vi "Read String in A.vi"(8 "error in (no error)":errorcluster, 11 "A in":refnum<class "A.lvclass">) -> (0 "error out":errorcluster, 2 "String in A":string, 3 "A out":refnum<class "A.lvclass">)   [LabVIEW 2013, in "A.lvclass"]
uses:
  A.lvclass
  A.lvclass/A.ctl
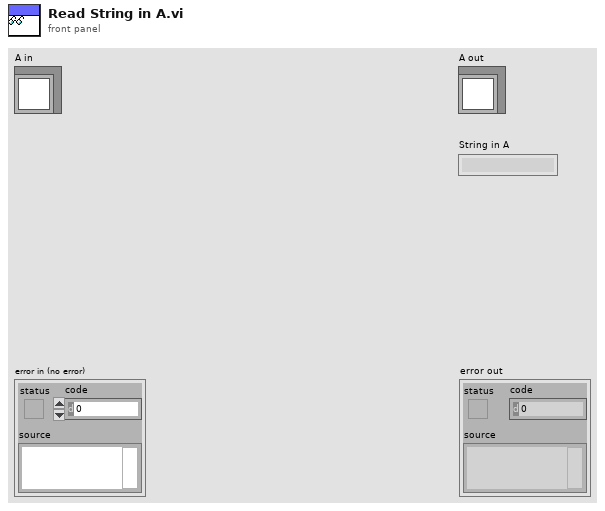
[diagram p1: front panel]
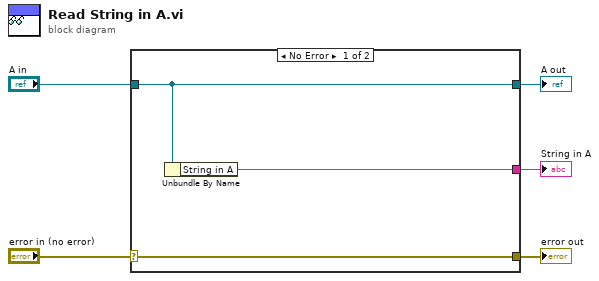
[diagram p0: block diagram]
diagram:
  n1 = case shown="No Error" "error in (no error)" {
    selector: "error in (no error)" -> [w8 w9]
    tunnel: [w8 w9] -> w4
    tunnel: [w7 w10] -> w2
    tunnel: "A in" -> [w7 w10]
    tunnel: [w6 _] -> w1
    frame No Error {
      n2 = Unbundle By Name(w7) -> ("String in A"=w6:string)
    }
    frame Error {
    }
  }
  "error out" <- w4
  "A out" <- w2
  "String in A" <- w1
